vi "Gaussian Peak Fit Intervals.vi"   [LabVIEW 2017, in "NI_AALPro.lvlib"]
doc: "Calculates statistical intervals of the best Gaussian fit for a data set (<B>X</B>, <B>Y</B>). You must manually select the polymorphic instance to use."
uses:
  NI_AALPro.lvlib
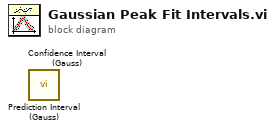
[diagram p0: block diagram]
diagram:
  n1 = call "Prediction Interval (Gauss).vi"() -> ()  [unwired: 13 in, 3 out]
  n2 = call "Confidence Interval (Gauss).vi"() -> ()  [unwired: 10 in, 6 out]
